vi "get_enum.vi"(11 "path":string) -> (0 "error out":errorcluster, 3 "Enum Elements":string[](array[string]))   [LabVIEW 2026]
doc: "Returns the elements of an enum stored in a .ctl file specified by path. Use this to see which elements a type-defined enum has."
uses:
  G-AI Core.lvlib
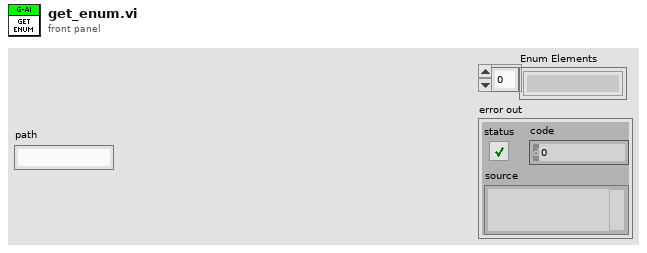
[diagram p1: front panel]
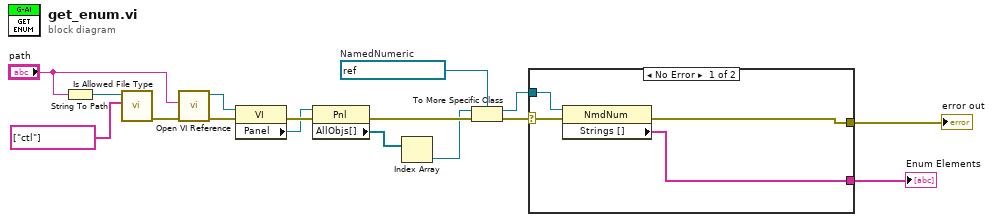
[diagram p0: block diagram]
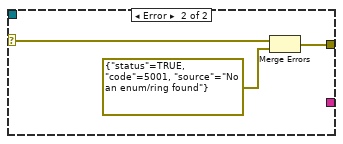
[diagram p2: hidden frame]
diagram:
  w8 = refnum<vi> refnum  # NamedNumeric
  n1 = String To Path(string="path") -> (path=w4:path)
  n2 = call "Is Allowed File Type.vi"("y"=string[] ["ctl"], "Path"=w4) -> ("error out"=w3:errorcluster)  [unwired: 9 in]
  n3 = call "Open VI Reference.vi"("error in"=w3, "VI Path"="path") -> ("error out"=w16:errorcluster, "VI Refnum"=w15:refnum<vi>)  [unwired: 8 in]
  n4 = property class="VI"(reference=w15, error in=w16) -> (error out=w14:errorcluster, "Panel"=w13:refnum<vi>)  [unwired: 1 out]
  n5 = property class="Pnl"(reference=w13, error in=w14) -> (error out=w11:errorcluster, "AllObjs[]"=w12:refnum<vi>[])  [unwired: 1 out]
  n6 = Index Array(array=w12) -> (element=w10:refnum<vi>)  [unwired: 1 in]
  n7 = To More Specific Class(target class=w8, reference=w10, error in=w11) -> (specific class reference=w9:refnum<vi>, error out=w5:errorcluster)
  n8 = case shown="No Error" w5 {
    selector: w5 -> [w17 w21]
    tunnel: w9 -> [w20 _]
    tunnel: [w19 _] -> w7
    tunnel: [w18 w22] -> w6
    frame No Error {
      n9 = property class="NmdNum"(reference=w20, error in=w17) -> (error out=w18:errorcluster, "Strings []"=w19:string[])  [unwired: 1 out]
    }
    frame Error {
      n10 = Merge Errors(w21, errorcluster {"status"=TRUE, "code"=5001, "source"="No an enum/ring found"} ("error out")) -> (w22:errorcluster)
    }
  }
  "Enum Elements" <- w7
  "error out" <- w6
